vi "auto arrived at setpoint.vi"(1 "Encoder Distance":dbl, 2 "Tolerance":dbl=0.05, 3 "Setpoint":dbl) -> (0 "At Location?":bool)   [LabVIEW 2014]
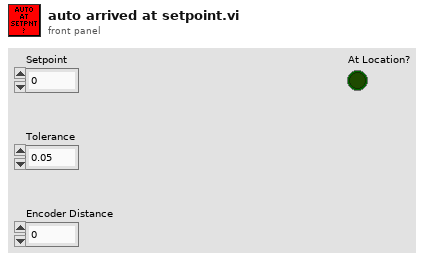
[diagram p1: front panel]
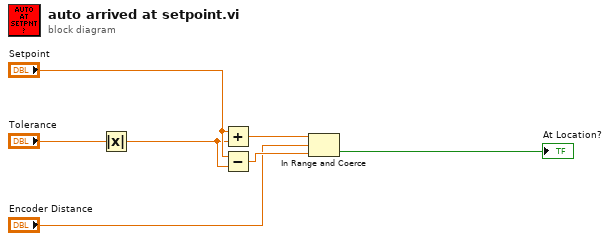
[diagram p0: block diagram]
diagram:
  n1 = Absolute Value(x="Tolerance") -> (abs(x)=w4:dbl)
  n2 = Add(x="Setpoint", y=w4) -> (x+y=w6:dbl)
  n3 = Subtract(x="Setpoint", y=w4) -> (x-y=w3:dbl)
  n4 = In Range and Coerce(upper limit=w6, x="Encoder Distance", lower limit=w3) -> (In Range?=→"At Location?":bool)  [unwired: 1 out]
